vi "testExample _GetPort.vi"(8 "error in (no error)":errorcluster, 11 "TestCase in":refnum<class "MyTestCase_shido.lvclass">) -> (0 "error out":errorcluster, 3 "TestCase out":refnum<class "MyTestCase_shido.lvclass">)   [LabVIEW 2020, in "MyTestCase_shido.lvclass"]
uses:
  MyTestCase_shido.lvclass
  Implementacion/Simulated/Simulated.lvclass
  <vilib>/addons/_JKI Toolkits/VI Tester/TestCase.llb/TestCase.lvclass
  C:/Program Files/National Instruments/LabVIEW 2020/vi.lib/addons/_JKI Toolkits/VI Tester/TestCase.llb/TestCase.lvclass
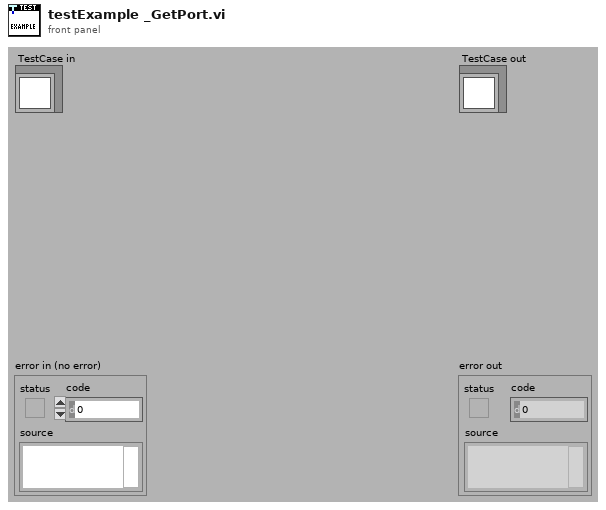
[diagram p1: front panel]
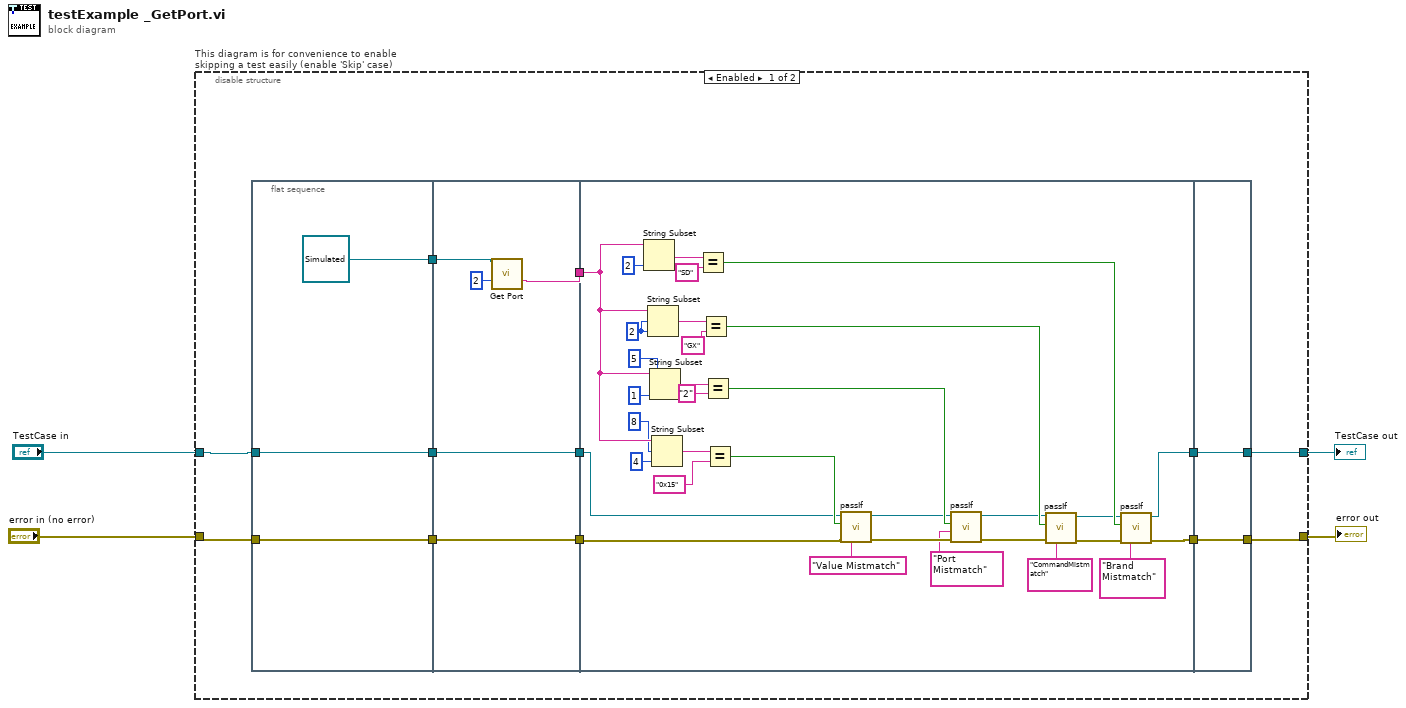
[diagram p0: block diagram]
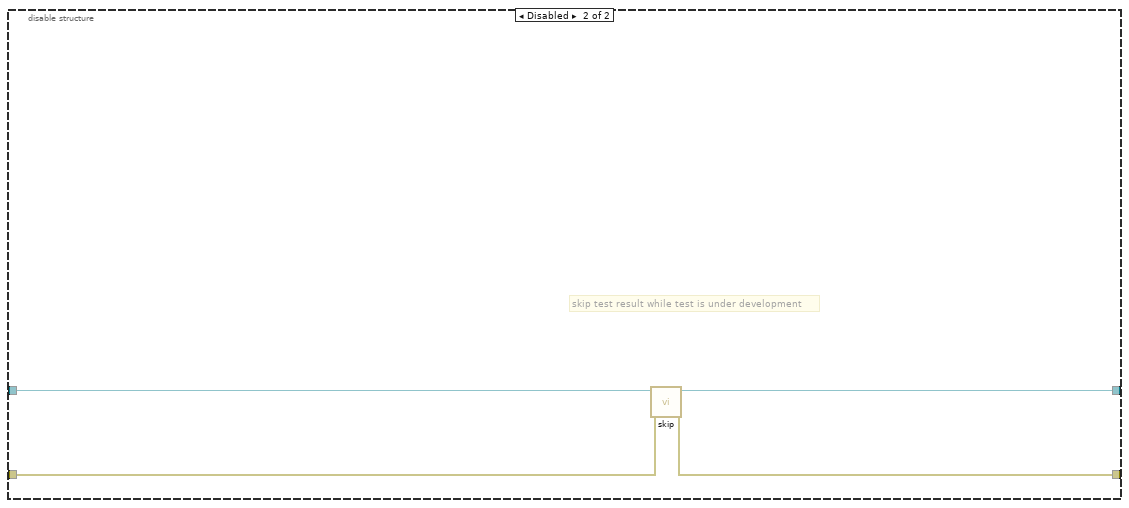
[diagram p2: hidden frame]
diagram:
  n1 = disable-structure "This diagram is for convenience to enable skipping a test easily (enable 'Skip' case)" shown="Enabled" {
    disable-tunnel: "TestCase in" -> [w8 w63]
    disable-tunnel: [w6 w61] -> w1
    disable-tunnel: [w5 w62] -> w3
    disable-tunnel: "error in (no error)" -> [w7 w60]
    frame Enabled {
      n2 = flat-sequence {
        tunnel: w8 -> [w17]
        tunnel: w7 -> [w18]
        tunnel: [refnum<class "Simulated.lvclass"> refnum ("Simulated.lvclass")] -> w16
        tunnel: [w18] -> w15
        tunnel: [w17] -> w14
        tunnel: w16 -> [w22]
        tunnel: [w21] -> w13
        tunnel: w15 -> [w24]
        tunnel: [w24] -> w12
        tunnel: w14 -> [w23]
        tunnel: [w23] -> w11
        tunnel: w13 -> [w47]
        tunnel: w12 -> [w34]
        tunnel: [w42] -> w10
        tunnel: [w29] -> w9
        tunnel: w11 -> [w25]
        tunnel: [w59] -> w5
        tunnel: w10 -> [w59]
        tunnel: w9 -> [w58]
        tunnel: [w58] -> w6
        frame #0 {
        }
        frame #1 {
          n3 = call-dynamic "Get Port.vi"("Simulated in"=w22, "Puerto"=u8 2) -> ("Response"=w21:string)  [unwired: 9 in, 4 out]
        }
        frame #2 {
          w54 = 2 ("length (rest)")
          n4 = String Subset(string=w47, length (rest)=2 ("length (rest)")) -> (substring=w56:string)  [unwired: 1 in]
          n5 = String Subset(string=w47, offset (0)=w54, length (rest)=w54) -> (substring=w53:string)
          n6 = String Subset(string=w47, offset (0)=5, length (rest)=1 ("length (rest)")) -> (substring=w48:string)
          n7 = String Subset(string=w47, offset (0)=8, length (rest)=4 ("length (rest)")) -> (substring=w44:string)
          n8 = Equal?(x=w56, y="SD") -> (x = y?=w41:bool)
          n9 = Equal?(x=w53, y="GX") -> (x = y?=w38:bool)
          n10 = Equal?(x=w48, y="2") -> (x = y?=w35:bool)
          n11 = Equal?(x=w44, y="0x15") -> (x = y?=w32:bool)
          n12 = call-dynamic "passIf.vi"("error in (no error)"=w34, "message (\"\")"="Value Mistmatch" ("message (\"\")"), "pass"=w32, "TestCase in"=w25) -> ("error out"=w33:errorcluster, "TestCase out"=w26:refnum<class "MyTestCase_shido.lvclass">)  [unwired: 6 in]
          n13 = call-dynamic "passIf.vi"("error in (no error)"=w33, "message (\"\")"="Port Mistmatch" ("message (\"\")"), "pass"=w35, "TestCase in"=w26) -> ("error out"=w36:errorcluster, "TestCase out"=w27:refnum<class "MyTestCase_shido.lvclass">)  [unwired: 6 in]
          n14 = call-dynamic "passIf.vi"("error in (no error)"=w36, "message (\"\")"="CommandMistmatch" ("message (\"\")"), "pass"=w38, "TestCase in"=w27) -> ("error out"=w39:errorcluster, "TestCase out"=w28:refnum<class "MyTestCase_shido.lvclass">)  [unwired: 6 in]
          n15 = call-dynamic "passIf.vi"("error in (no error)"=w39, "message (\"\")"="Brand Mistmatch" ("message (\"\")"), "pass"=w41, "TestCase in"=w28) -> ("error out"=w42:errorcluster, "TestCase out"=w29:refnum<class "MyTestCase_shido.lvclass">)  [unwired: 6 in]
        }
        frame #3 {
        }
      }
    }
    frame Disabled {
      # "skip test result while test is under development"
      n16 = call <vilib>:"skip.vi"("error in (no error)"=w60, "TestCase in"=w63) -> ("error out"=w62:errorcluster, "TestCase out"=w61:refnum<class "MyTestCase_shido.lvclass">)  [unwired: 8 in]
    }
  }
  "error out" <- w3
  "TestCase out" <- w1
